vi "HEWH Find End of Draw.vi"(8 "Error In":errorcluster, 10 "UEF Calculated Values":T1={"Calculated Values"={"Draw Cluster - Actual (Gal)"=[], "Tdel_actual - Outlet Draw Cluster (°F)"=[], "Tin - Inlet Draw Cluster (°F)"=[], "Mass of water All (lbm)"=[], "Density of hot water All (lbm/gal)"=[], "CpHW (BTU/(lbm °F))"=[], "QHW (BTU)"=[], "QHWD (BTU)"=[], "Qdm (BTU)"=[], "rho 2 (lb/gal)"=0.0, "rho standby (lb/gal)"=0.0, "rho 24 (lb/gal)"=0.0, "Cp1 (BTU/(lb*F))"=0.0, "Cp2 (BTU/(lb*F))"=0.0, "Cp standby (BTU/(lb*F))"=0.0, "Cp 24 (BTU/(lb*F))"=0.0, "CpUEF (BTU/(lb*F))"=0.0, "nu_r"=0.0, "Qstby (BTU)"=0.0, "Qhr (BTU/hr)"=0.0, "UA (BTU/(hr*F))"=0.0, "Q (BTU)"=0.0, "Qd (BTU)"=0.0, "Qda (BTU)"=0.0, "QHW67 (BTU)"=0.0, "UEF"=0.0, "Tdel1 - Mean Outlet 1st Cluster (°F)"=0.0, "Tin1 - Mean Inlet 1st Cluster (°F)"=0.0, "rho theoretical (lbm/gal)"=0.0, "Cp theoretical (BTU/(lbm °F))"=0.0, "M cluster mass removed (lbm)"=0.0, "M all mass removed (lbm)"=0.0}, "Sampled Data"={"Draw Amounts - Actual (Gal)"=[14.98, 1.97, 9.0, 8.97, 4.98, 0.98, 0.96, 0.96, 0.96, 1.96, 1.99, 6.98], "T del_all - Outlet Temps (°F)"=[121.5, 121.3, 124.5, 120.0, 121.2, 120.1, 119.0, 120.3, 116.6, 118.8, 118.3, 118.3], "T in_all - Inlet Temps (°F)"=[58.5, 58.2, 58.4, 58.6, 58.6, 58.1, 58.1, 58.3, 56.3, 58.5, 58.5, 58.5], "Qsu0 (BTU)"=9772.3, "Qsuf (BTU)"=9773.0, "Tau stby_1 (hr)"=6.7, "T suf(°F)"=107.7, "T su0(°F)"=109.3, "T tstby(°F)"=108.5, "T astby(°F)"=68.2, "T 24(°F)"=117.9, "Qr (BTU)"=7628.5, "T0 (°F)"=121.1, "Tmax1 (°F)"=122.4, "Qe (BTU)"=29606.3, "Qf (BTU)"=0.0, "Tastby2 (°F)"=68.3}, "Static Data"={"T-Wh Setpoint (°F)"=125.0, "T-Inlet Setpoint (°F)"=58.0, "T-Ambinet Nominal (°F)"=67.5, "V - Volume of Wh (True)"=46.0, "Tau stby2 (hr)"=23.406}, "Data Indexes"={"T0 Index"=0, "Header Length"=0, "End of First Draw Index"=0, "Draw Index Array"=[], "First Recovery Start"=0, "First Recovery End"=0, "Start Watt Hours"=0.0, "Tsu Index"=0, "End of First Cluster"=0, "Next Draw Start (After 1st Cluster)"=0, "Tsf Index"=0}} {"Static Data"."Tau stby2 (hr)" format="%#.3f"; "Static Data"."V - Volume of Wh (True)" format="%#.3f"; "Static Data"."T-Ambinet Nominal (°F)" format="%#.3f"; "Static Data"."T-Inlet Setpoint (°F)" format="%#.3f"; "Static Data"."T-Wh Setpoint (°F)" format="%#.3f"; "Sampled Data"."Tastby2 (°F)" format="%#.3f"; "Sampled Data"."Qf (BTU)" format="%#.3f"; "Sampled Data"."Qe (BTU)" format="%#.3f"; "Sampled Data"."Tmax1 (°F)" format="%#.3f"; "Sampled Data"."T0 (°F)" format="%#.3f"; "Sampled Data"."Qr (BTU)" format="%#.3f"; "Sampled Data"."T 24(°F)" format="%#.3f"; "Sampled Data"."T astby(°F)" format="%#.3f"; "Sampled Data"."T tstby(°F)" format="%#.3f"; "Sampled Data"."T su0(°F)" format="%#.3f"; "Sampled Data"."T suf(°F)" format="%#.3f"; "Sampled Data"."Tau stby_1 (hr)" format="%#.3f"; "Sampled Data"."Qsuf (BTU)" format="%#.3f"; "Sampled Data"."Qsu0 (BTU)" format="%#.3f"; "Calculated Values"."M all mass removed (lbm)" format="%#.3f"; "Calculated Values"."M cluster mass removed (lbm)" format="%#.3f"; "Calculated Values"."Cp theoretical (BTU/(lbm °F))" format="%#.3f"; "Calculated Values"."rho theoretical (lbm/gal)" format="%#.3f"; "Calculated Values"."Tin1 - Mean Inlet 1st Cluster (°F)" format="%#.3f"; "Calculated Values"."Tdel1 - Mean Outlet 1st Cluster (°F)" format="%#.3f"; "Calculated Values"."UEF" format="%#.3f"; "Calculated Values"."QHW67 (BTU)" format="%#.3f"; "Calculated Values"."Qda (BTU)" format="%#.3f"; "Calculated Values"."Qd (BTU)" format="%#.3f"; "Calculated Values"."Q (BTU)" format="%#.3f"; "Calculated Values"."UA (BTU/(hr*F))" format="%#.3f"; "Calculated Values"."Qhr (BTU/hr)" format="%#.3f"; "Calculated Values"."Qstby (BTU)" format="%#.3f"; "Calculated Values"."nu_r" format="%#.3f"; "Calculated Values"."CpUEF (BTU/(lb*F))" format="%#.3f"; "Calculated Values"."Cp 24 (BTU/(lb*F))" format="%#.3f"; "Calculated Values"."Cp standby (BTU/(lb*F))" format="%#.3f"; "Calculated Values"."Cp2 (BTU/(lb*F))" format="%#.3f"; "Calculated Values"."Cp1 (BTU/(lb*F))" format="%#.3f"; "Calculated Values"."rho 24 (lb/gal)" format="%#.3f"; "Calculated Values"."rho standby (lb/gal)" format="%#.3f"; "Calculated Values"."rho 2 (lb/gal)" format="%#.3f"; "Calculated Values"."Qdm (BTU)" format="%#.3f"; "Calculated Values"."QHWD (BTU)" format="%#.3f"; "Calculated Values"."QHW (BTU)" format="%#.3f"; "Calculated Values"."CpHW (BTU/(lbm °F))" format="%#.3g"; "Calculated Values"."Density of hot water All (lbm/gal)" format="%#.3g"; "Calculated Values"."Mass of water All (lbm)" format="%#.3f"}, 11 "Full Data Input":string[][](array[string])) -> (0 "Error Out":errorcluster, 2 "UEF Calculated Values Output":T1={"Calculated Values"={"Draw Cluster - Actual (Gal)"=[], "Tdel_actual - Outlet Draw Cluster (°F)"=[], "Tin - Inlet Draw Cluster (°F)"=[], "Mass of water All (lbm)"=[], "Density of hot water All (lbm/gal)"=[], "CpHW (BTU/(lbm °F))"=[], "QHW (BTU)"=[], "QHWD (BTU)"=[], "Qdm (BTU)"=[], "rho 2 (lb/gal)"=0.0, "rho standby (lb/gal)"=0.0, "rho 24 (lb/gal)"=0.0, "Cp1 (BTU/(lb*F))"=0.0, "Cp2 (BTU/(lb*F))"=0.0, "Cp standby (BTU/(lb*F))"=0.0, "Cp 24 (BTU/(lb*F))"=0.0, "CpUEF (BTU/(lb*F))"=0.0, "nu_r"=0.0, "Qstby (BTU)"=0.0, "Qhr (BTU/hr)"=0.0, "UA (BTU/(hr*F))"=0.0, "Q (BTU)"=0.0, "Qd (BTU)"=0.0, "Qda (BTU)"=0.0, "QHW67 (BTU)"=0.0, "UEF"=0.0, "Tdel1 - Mean Outlet 1st Cluster (°F)"=0.0, "Tin1 - Mean Inlet 1st Cluster (°F)"=0.0, "rho theoretical (lbm/gal)"=0.0, "Cp theoretical (BTU/(lbm °F))"=0.0, "M cluster mass removed (lbm)"=0.0, "M all mass removed (lbm)"=0.0}, "Sampled Data"={"Draw Amounts - Actual (Gal)"=[14.98, 1.97, 9.0, 8.97, 4.98, 0.98, 0.96, 0.96, 0.96, 1.96, 1.99, 6.98], "T del_all - Outlet Temps (°F)"=[121.5, 121.3, 124.5, 120.0, 121.2, 120.1, 119.0, 120.3, 116.6, 118.8, 118.3, 118.3], "T in_all - Inlet Temps (°F)"=[58.5, 58.2, 58.4, 58.6, 58.6, 58.1, 58.1, 58.3, 56.3, 58.5, 58.5, 58.5], "Qsu0 (BTU)"=9772.3, "Qsuf (BTU)"=9773.0, "Tau stby_1 (hr)"=6.7, "T suf(°F)"=107.7, "T su0(°F)"=109.3, "T tstby(°F)"=108.5, "T astby(°F)"=68.2, "T 24(°F)"=117.9, "Qr (BTU)"=7628.5, "T0 (°F)"=121.1, "Tmax1 (°F)"=122.4, "Qe (BTU)"=29606.3, "Qf (BTU)"=0.0, "Tastby2 (°F)"=68.3}, "Static Data"={"T-Wh Setpoint (°F)"=125.0, "T-Inlet Setpoint (°F)"=58.0, "T-Ambinet Nominal (°F)"=67.5, "V - Volume of Wh (True)"=46.0, "Tau stby2 (hr)"=23.406}, "Data Indexes"={"T0 Index"=0, "Header Length"=0, "End of First Draw Index"=0, "Draw Index Array"=[], "First Recovery Start"=0, "First Recovery End"=0, "Start Watt Hours"=0.0, "Tsu Index"=0, "End of First Cluster"=0, "Next Draw Start (After 1st Cluster)"=0, "Tsf Index"=0}} {"Static Data"."Tau stby2 (hr)" format="%#.3f"; "Static Data"."V - Volume of Wh (True)" format="%#.3f"; "Static Data"."T-Ambinet Nominal (°F)" format="%#.3f"; "Static Data"."T-Inlet Setpoint (°F)" format="%#.3f"; "Static Data"."T-Wh Setpoint (°F)" format="%#.3f"; "Sampled Data"."Tastby2 (°F)" format="%#.3f"; "Sampled Data"."Qf (BTU)" format="%#.3f"; "Sampled Data"."Qe (BTU)" format="%#.3f"; "Sampled Data"."Tmax1 (°F)" format="%#.3f"; "Sampled Data"."T0 (°F)" format="%#.3f"; "Sampled Data"."Qr (BTU)" format="%#.3f"; "Sampled Data"."T 24(°F)" format="%#.3f"; "Sampled Data"."T astby(°F)" format="%#.3f"; "Sampled Data"."T tstby(°F)" format="%#.3f"; "Sampled Data"."T su0(°F)" format="%#.3f"; "Sampled Data"."T suf(°F)" format="%#.3f"; "Sampled Data"."Tau stby_1 (hr)" format="%#.3f"; "Sampled Data"."Qsuf (BTU)" format="%#.3f"; "Sampled Data"."Qsu0 (BTU)" format="%#.3f"; "Calculated Values"."M all mass removed (lbm)" format="%#.3f"; "Calculated Values"."M cluster mass removed (lbm)" format="%#.3f"; "Calculated Values"."Cp theoretical (BTU/(lbm °F))" format="%#.3f"; "Calculated Values"."rho theoretical (lbm/gal)" format="%#.3f"; "Calculated Values"."Tin1 - Mean Inlet 1st Cluster (°F)" format="%#.3f"; "Calculated Values"."Tdel1 - Mean Outlet 1st Cluster (°F)" format="%#.3f"; "Calculated Values"."UEF" format="%#.3f"; "Calculated Values"."QHW67 (BTU)" format="%#.3f"; "Calculated Values"."Qda (BTU)" format="%#.3f"; "Calculated Values"."Qd (BTU)" format="%#.3f"; "Calculated Values"."Q (BTU)" format="%#.3f"; "Calculated Values"."UA (BTU/(hr*F))" format="%#.3f"; "Calculated Values"."Qhr (BTU/hr)" format="%#.3f"; "Calculated Values"."Qstby (BTU)" format="%#.3f"; "Calculated Values"."nu_r" format="%#.3f"; "Calculated Values"."CpUEF (BTU/(lb*F))" format="%#.3f"; "Calculated Values"."Cp 24 (BTU/(lb*F))" format="%#.3f"; "Calculated Values"."Cp standby (BTU/(lb*F))" format="%#.3f"; "Calculated Values"."Cp2 (BTU/(lb*F))" format="%#.3f"; "Calculated Values"."Cp1 (BTU/(lb*F))" format="%#.3f"; "Calculated Values"."rho 24 (lb/gal)" format="%#.3f"; "Calculated Values"."rho standby (lb/gal)" format="%#.3f"; "Calculated Values"."rho 2 (lb/gal)" format="%#.3f"; "Calculated Values"."Qdm (BTU)" format="%#.3f"; "Calculated Values"."QHWD (BTU)" format="%#.3f"; "Calculated Values"."QHW (BTU)" format="%#.3f"; "Calculated Values"."CpHW (BTU/(lbm °F))" format="%#.3g"; "Calculated Values"."Density of hot water All (lbm/gal)" format="%#.3g"; "Calculated Values"."Mass of water All (lbm)" format="%#.3f"}, 3 "Full Data Output":string[][](array[string]))   [LabVIEW 2016]
uses:
  Type Definitions/UEF Constants.ctl
  Type Definitions/HEWH Draw Stats.ctl
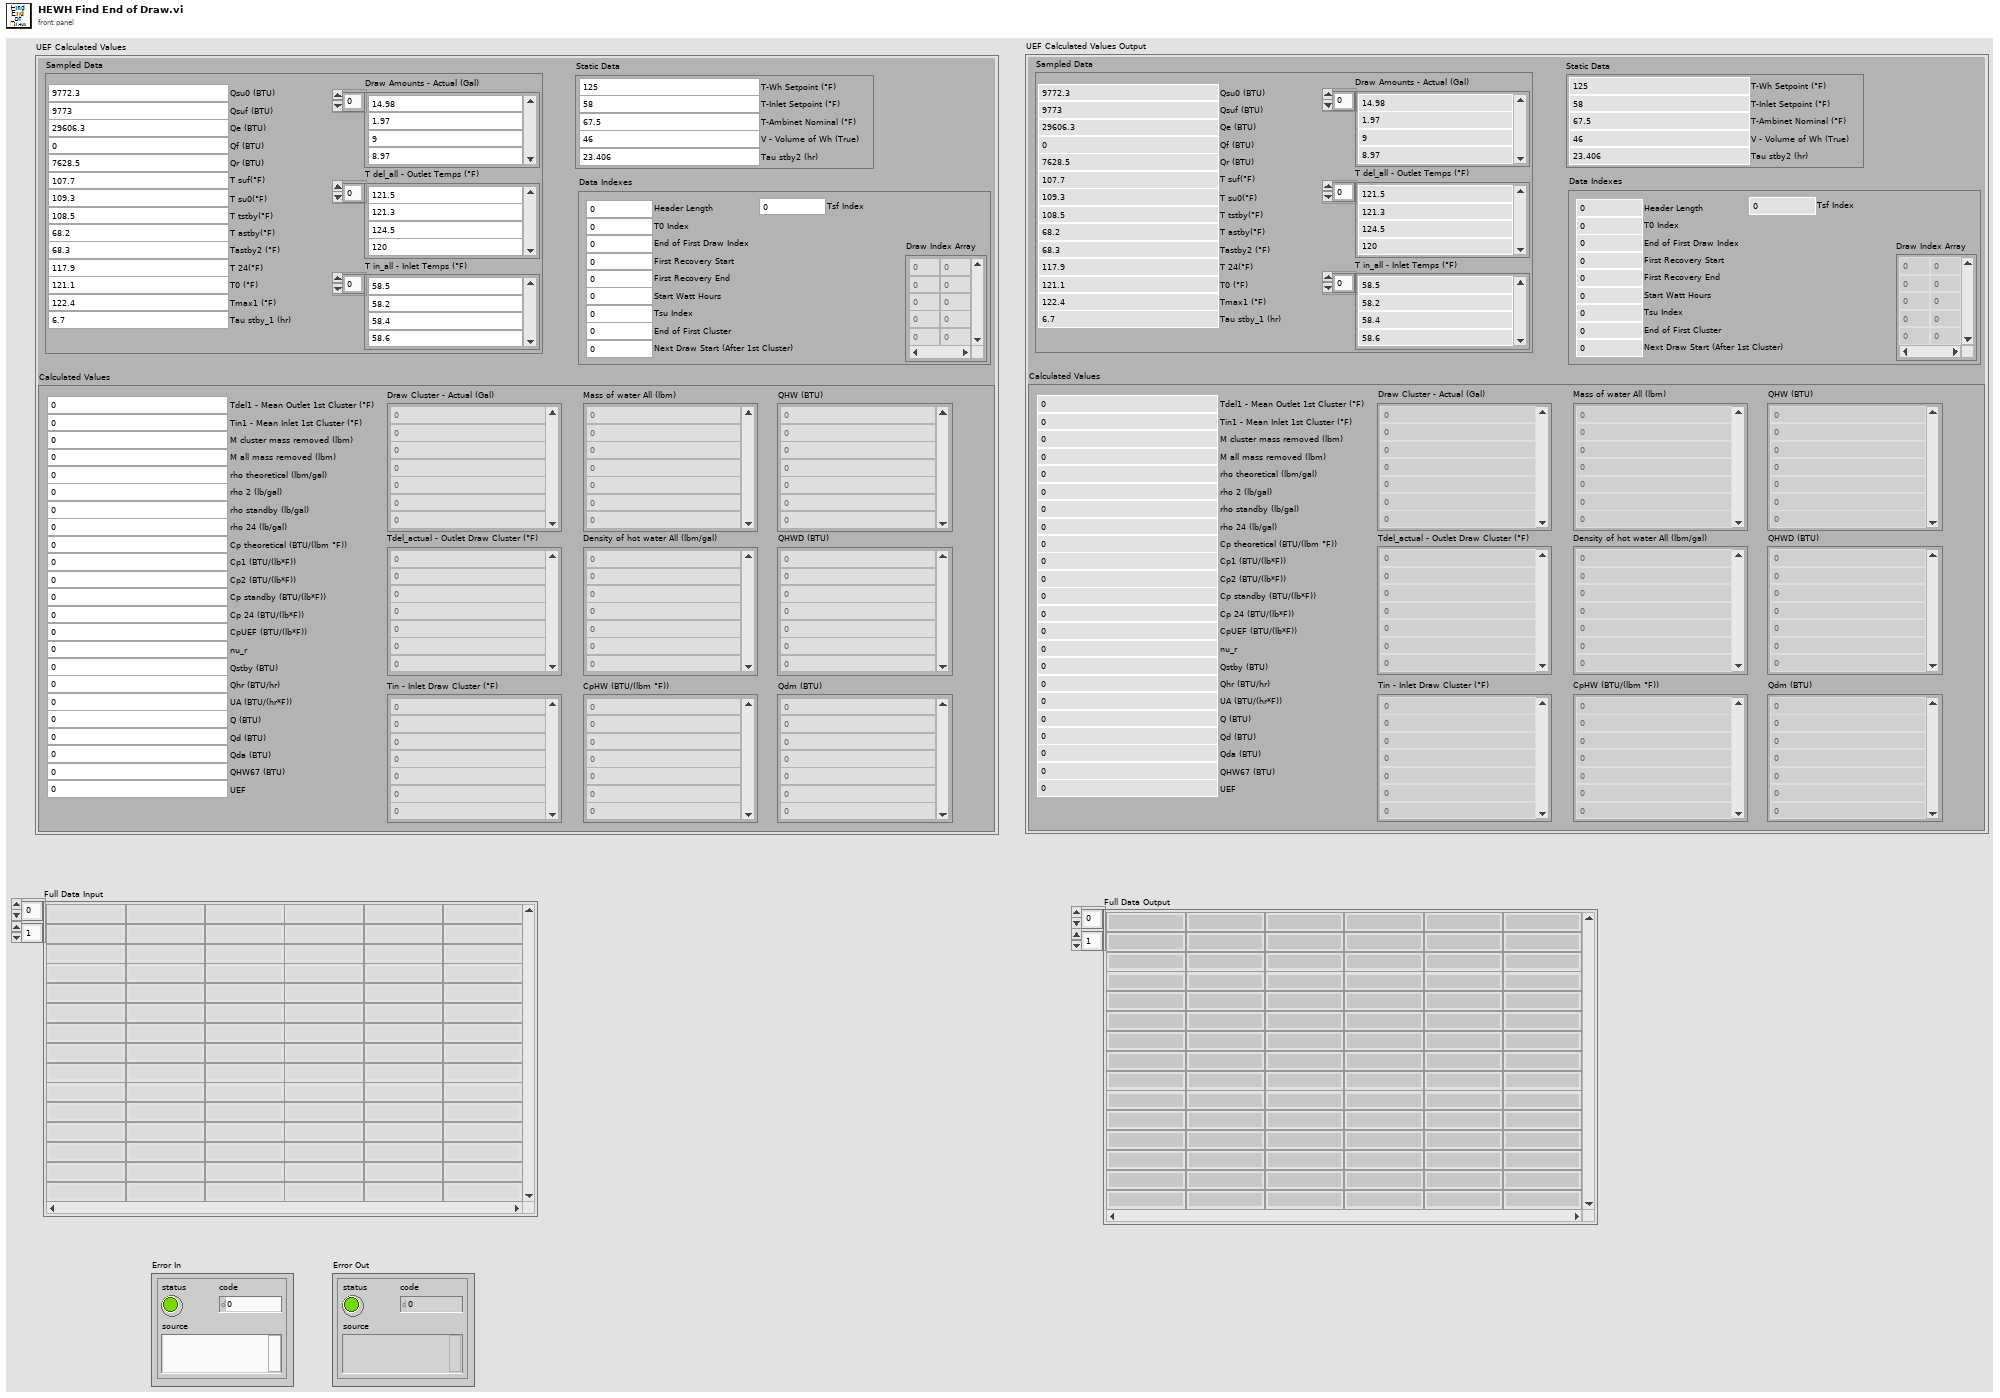
[diagram p1: front panel]
types:
  T1 = typedef "UEF Constants.ctl" = cluster{"Calculated Values":T2, "Sampled Data":cluster{"Draw Amounts - Actual (Gal)":dbl[], "T del_all - Outlet Temps (°F)":dbl[], "T in_all - Inlet Temps (°F)":dbl[], "Qsu0 (BTU)":dbl, "Qsuf (BTU)":dbl, "Tau stby_1 (hr)":dbl, "T suf(°F)":dbl, "T su0(°F)":dbl, "T tstby(°F)":dbl, "T astby(°F)":dbl, "T 24(°F)":dbl, "Qr (BTU)":dbl, "T0 (°F)":dbl, "Tmax1 (°F)":dbl, "Qe (BTU)":dbl, "Qf (BTU)":dbl, "Tastby2 (°F)":dbl}, "Static Data":cluster{"T-Wh Setpoint (°F)":dbl, "T-Inlet Setpoint (°F)":dbl, "T-Ambinet Nominal (°F)":dbl, "V - Volume of Wh (True)":dbl, "Tau stby2 (hr)":dbl}, "Data Indexes":cluster{"T0 Index":i32, "Header Length":i32, "End of First Draw Index":i32, "Draw Index Array":i32[][], "First Recovery Start":i32, "First Recovery End":i32, "Start Watt Hours":dbl, "Tsu Index":i32, "End of First Cluster":i32, "Next Draw Start (After 1st Cluster)":i32, "Tsf Index":i32}}
  T2 = typedef "HEWH Draw Stats.ctl" = cluster{"Draw Cluster - Actual (Gal)":dbl[], "Tdel_actual - Outlet Draw Cluster (°F)":dbl[], "Tin - Inlet Draw Cluster (°F)":dbl[], "Mass of water All (lbm)":dbl[], "Density of hot water All (lbm/gal)":dbl[], "CpHW (BTU/(lbm °F))":dbl[], "QHW (BTU)":dbl[], "QHWD (BTU)":dbl[], "Qdm (BTU)":dbl[], "rho 2 (lb/gal)":dbl, "rho standby (lb/gal)":dbl, "rho 24 (lb/gal)":dbl, "Cp1 (BTU/(lb*F))":dbl, "Cp2 (BTU/(lb*F))":dbl, "Cp standby (BTU/(lb*F))":dbl, "Cp 24 (BTU/(lb*F))":dbl, "CpUEF (BTU/(lb*F))":dbl, "nu_r":dbl, "Qstby (BTU)":dbl, "Qhr (BTU/hr)":dbl, "UA (BTU/(hr*F))":dbl, "Q (BTU)":dbl, "Qd (BTU)":dbl, "Qda (BTU)":dbl, "QHW67 (BTU)":dbl, "UEF":dbl, "Tdel1 - Mean Outlet 1st Cluster (°F)":dbl, "Tin1 - Mean Inlet 1st Cluster (°F)":dbl, "rho theoretical (lbm/gal)":dbl, "Cp theoretical (BTU/(lbm °F))":dbl, "M cluster mass removed (lbm)":dbl, "M all mass removed (lbm)":dbl}
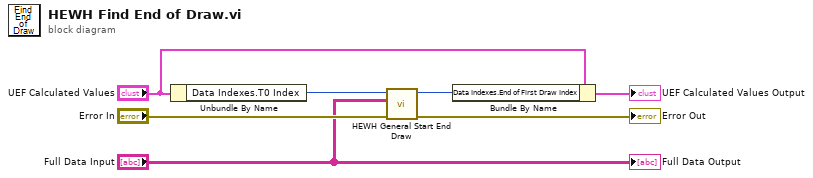
[diagram p0: block diagram]
diagram:
  n1 = Unbundle By Name("UEF Calculated Values") -> ("Data Indexes.T0 Index"=w4:i32)
  n2 = call "HEWH General Start End Draw.vi"("error in (no error)"="Error In", "Full Data Input"="Full Data Input", "Start Index"=w4) -> ("error out"=→"Error Out":errorcluster, "End Index"=w2:i32)  [unwired: 7 in]
  n3 = Bundle By Name(cluster="UEF Calculated Values", "Data Indexes.End of First Draw Index"=w2) -> (→"UEF Calculated Values Output":T1)
  "Full Data Output" <- "Full Data Input"
